vi "2039_hw INAVGetData.vi"(3 "Rightward Direction":T1(ring), 4 "Forward Direction":enum16{"X Forward", "Y Forward", "Z Forward"}(ring), 5 "INAV Sensor Cluster":T11 {"GyroDevRef"."Sample Rate" min=0.25 max=100.0 step=0.25; "AccelerometerDevRef"."Device Address" format="%.0x"; "AccelerometerDevRef"."Accel Range" items=["+/- 2 g", "+/- 4 g", "+/- 8 g", "+/- 16 g"]}) -> (0 "Rightward Accel":dbl, 1 "Forward Accel":dbl, 2 "INAV Sensor Cluster":T11 {"GyroDevRef"."Sample Rate" min=0.25 max=100.0 step=0.25; "AccelerometerDevRef"."Device Address" format="%.0x"; "AccelerometerDevRef"."Accel Range" items=["+/- 2 g", "+/- 4 g", "+/- 8 g", "+/- 16 g"]})   [LabVIEW 2016, in "2039lib.lvlib"]
uses:
  2039lib.lvlib
  <vilib>/Rock Robotics/WPI/Gyro/WPI_GyroDevRef.ctl
  <vilib>/Rock Robotics/SystemInterfaces/AI/FPGA_AIChannel.ctl
  <vilib>/Rock Robotics/SystemInterfaces/spilib/spi_bus.ctl
  <vilib>/Rock Robotics/WPI/Accelerometer/WPI_AccelerometerDevRef.ctl
  <vilib>/Rock Robotics/WPI/Accelerometer/WPI_AccelerometerScaling.ctl
  <vilib>/Rock Robotics/WPI/Accelerometer/WPI_AccelerometerAnalogChannels.ctl
  <vilib>/Rock Robotics/SystemInterfaces/i2clib/i2c_bus.ctl
  <vilib>/Rock Robotics/WPI/Accelerometer/ADXL345 Range.ctl
  <vilib>/Rock Robotics/WPI/Accelerometer/WPI_AccelerometerADXL345 Axes.ctl
panel:
  # "Analog"
  # "XRS"
  # "ADXL"
  # "Analog"
  # "Analog"
  # "XRS"
  # "ADXL"
  # "Analog"
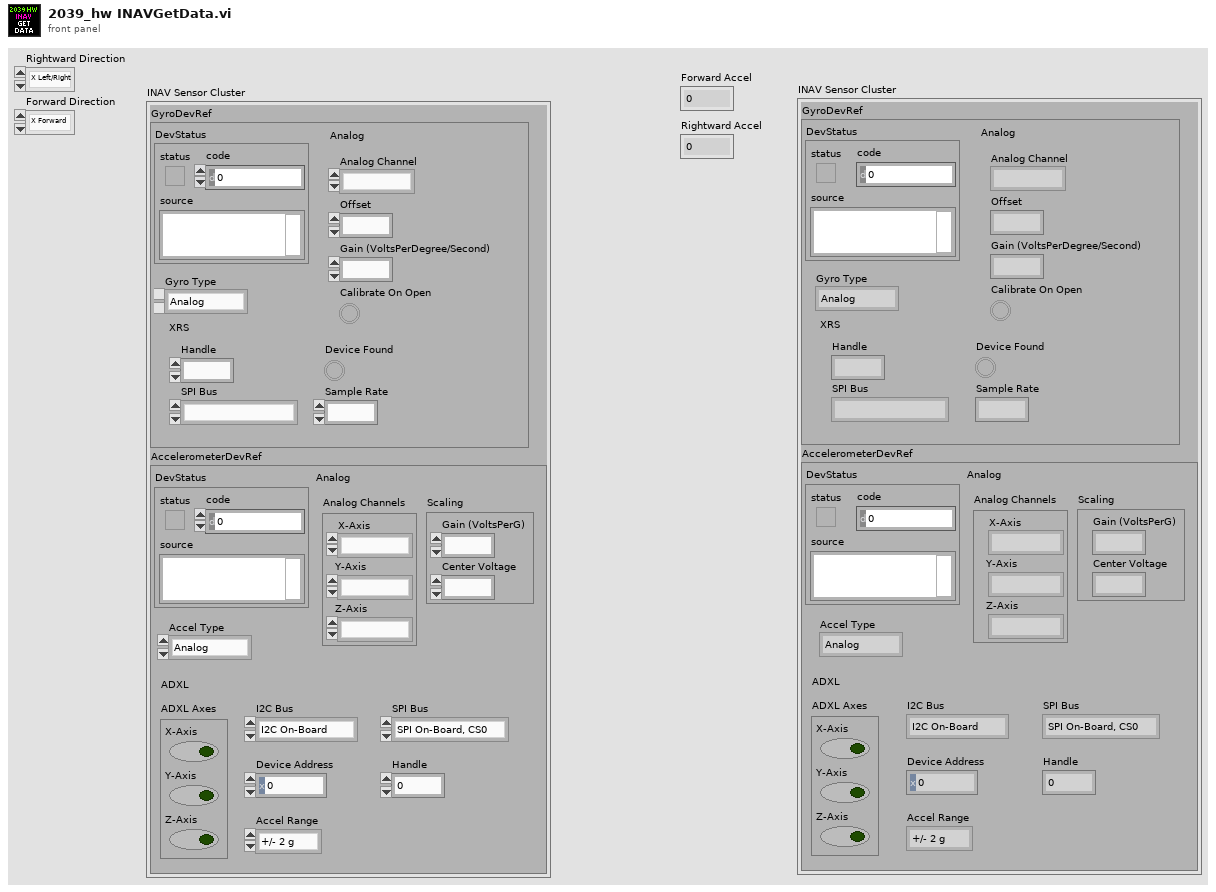
[diagram p1: front panel]
types:
  T1 = enum16{"X Left/Right", "Y Left/Right", "Z Left/Right"}
  T2 = typedef "WPI_GyroDevRef.ctl" = cluster{"DevStatus":errorcluster, "Analog Channel":T3, "Offset":dbl, "Gain (VoltsPerDegree/Second)":dbl, "Gyro Type":enum16{"Analog", "XRS450"}, "Handle":i32, "SPI Bus":T4, "Device Found":bool, "Sample Rate":dbl, "Calibrate On Open":bool}
  T3 = typedef "FPGA_AIChannel.ctl" = enum8{"AI 0", "AI 1", "AI 2", "AI 3", "AI MXP 0", "AI MXP 1", "AI MXP 2", "AI MXP 3", "Invalid"}
  T4 = typedef "spi_bus.ctl" = enum16{"SPI On-Board, CS0", "SPI On-Board, CS1", "SPI On-Board, CS2", "SPI On-Board, CS3", "SPI MXP", "Invalid"}
  T5 = typedef "WPI_AccelerometerDevRef.ctl" = cluster{"DevStatus":errorcluster, "Scaling":T6, "Analog Channels":T7, "I2C Bus":T8, "SPI Bus":T4, "Accel Range":T9, "ADXL Axes":T10, "Handle":i32, "Device Address":u8, "Accel Type":enum16{"Analog", "ADXL345 I2C", "ADXL345 SPI", "Internal", "ADXL362 SPI"}}
  T6 = typedef "WPI_AccelerometerScaling.ctl" = cluster{"Gain (VoltsPerG)":dbl, "Center Voltage":dbl}
  T7 = typedef "WPI_AccelerometerAnalogChannels.ctl" = cluster{"X-Axis":T3, "Y-Axis":T3, "Z-Axis":T3}
  T8 = typedef "i2c_bus.ctl" = enum16{"I2C On-Board", "I2C MXP", "Invalid"}
  T9 = typedef "ADXL345 Range.ctl" = u8
  T10 = typedef "WPI_AccelerometerADXL345 Axes.ctl" = cluster{"X-Axis":bool, "Y-Axis":bool, "Z-Axis":bool}
  T11 = cluster{"GyroDevRef":T2, "AccelerometerDevRef":T5}
  T12 = cluster{"X-Axis":dbl, "Y-Axis":dbl, "Z-Axis":dbl}
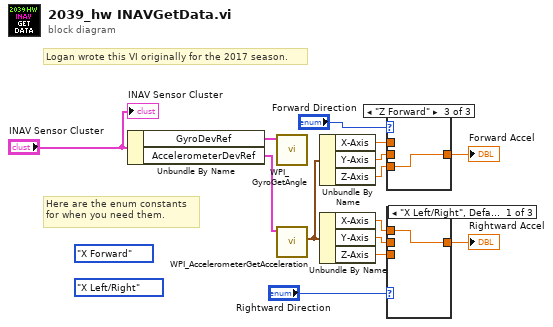
[diagram p0: block diagram]
diagram:
  (unwired) T1."X Left/Right"
  (unwired) enum16{"X Forward", "Y Forward", "Z Forward"}."X Forward"
  # "Logan wrote this VI originally for the 2017 season."
  # "Here are the enum constants\nfor when you need them."
  n1 = Unbundle By Name("INAV Sensor Cluster") -> ("GyroDevRef"=w13:T2, "AccelerometerDevRef"=w14:T5)
  n2 = call <vilib>:"WPI_GyroGetAngle.vi"("GyroDevRef"=w13) -> ()  [unwired: 7 in, 4 out]
  n3 = call <vilib>:"WPI_AccelerometerGetAcceleration.vi"("AccelerometerDevRef"=w14) -> ("Accelerations"=w7:T12)  [unwired: 8 in, 2 out]
  n4 = Unbundle By Name(w7) -> ("X-Axis"=w11:dbl, "Y-Axis"=w10:dbl, "Z-Axis"=w9:dbl)
  n5 = Unbundle By Name(w7) -> ("X-Axis"=w6:dbl, "Y-Axis"=w4:dbl, "Z-Axis"=w3:dbl)
  n6 = case shown="\"Z Forward\"" "Forward Direction" {
    tunnel: w11 -> [w15 _ _]
    tunnel: w10 -> [_ w16 _]
    tunnel: w9 -> [_ _ w17]
    tunnel: [w15 w16 w17] -> w8
    frame "X Forward", Default {
    }
    frame "Y Forward" {
    }
    frame "Z Forward" {
    }
  }
  "Forward Accel" <- w8
  n7 = case shown="\"X Left/Right\", Default" "Rightward Direction" {
    tunnel: w6 -> [w18 _ _]
    tunnel: [w18 w19 w20] -> w5
    tunnel: w4 -> [_ w19 _]
    tunnel: w3 -> [_ _ w20]
    frame "X Left/Right", Default {
    }
    frame "Y Left/Right" {
    }
    frame "Z Left/Right" {
    }
  }
  "Rightward Accel" <- w5
  "INAV Sensor Cluster" <- "INAV Sensor Cluster"
